vi "VI_Info_do_Robô_Dashboard.vi"() -> (1 "Autonomous":string, 2 "March_Indicator":dbl, 3 "Elevator_Indicator":string)   [LabVIEW 2017]
uses:
  <vilib>/Rock Robotics/Network Tables/NT Read Number.vi
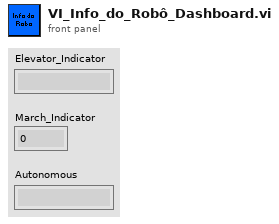
[diagram p1: front panel]
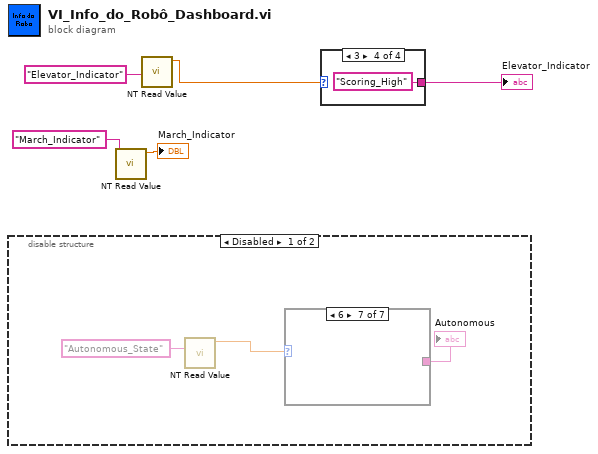
[diagram p0: block diagram]
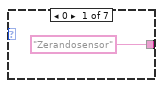
[diagram p2: hidden frame]
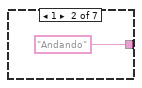
[diagram p3: hidden frame]
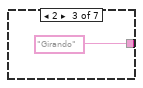
[diagram p4: hidden frame]
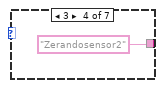
[diagram p5: hidden frame]
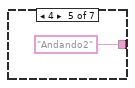
[diagram p6: hidden frame]
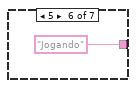
[diagram p7: hidden frame]
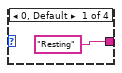
[diagram p9: hidden frame]
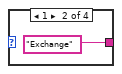
[diagram p10: hidden frame]
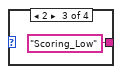
[diagram p11: hidden frame]
diagram:
  n1 = disable-structure shown="Disabled" {
    frame Disabled {
      n2 = call-poly <vilib>:"NT Read Value.vi"("Name"="Autonomous_State") -> ("Numeric"=w7:dbl)  [unwired: 9 in, 1 out]
      n3 = case shown="6" w7 {
        tunnel: ["Zerandosensor" "Andando" "Girando" "Zerandosensor2" "Andando2" "Jogando" _] -> w6
        frame 0 {
        }
        frame 1 {
        }
        frame 2 {
        }
        frame 3 {
        }
        frame 4 {
        }
        frame 5 {
        }
        frame 6 {
        }
      }
      "Autonomous" <- w6
    }
    frame Enabled {
    }
  }
  n4 = call-poly <vilib>:"NT Read Value.vi"("Name"="March_Indicator") -> ("Numeric"=→"March_Indicator":dbl)  [unwired: 9 in, 1 out]
  n5 = call-poly <vilib>:"NT Read Value.vi"("Name"="Elevator_Indicator") -> ("Numeric"=w2:dbl)  [unwired: 9 in, 1 out]
  n6 = case shown="3" w2 {
    tunnel: ["Resting" "Exchange" "Scoring_Low" "Scoring_High"] -> w1
    frame 0, Default {
    }
    frame 1 {
    }
    frame 2 {
    }
    frame 3 {
    }
  }
  "Elevator_Indicator" <- w1
